vi "test_Delete FPGA Addon.vi"(8 "error in (no error)":errorcluster, 11 "TestCase in":refnum<class "FPGA Addon Scripting API Unit Tests.lvclass">) -> (0 "error out":errorcluster, 3 "TestCase out":refnum<class "FPGA Addon Scripting API Unit Tests.lvclass">)   [LabVIEW 2021, in "FPGA Addon Scripting API Unit Tests.lvclass"]
uses:
  FPGA Addon Scripting API Unit Tests.lvclass
  <vilib>/addons/_JKI Toolkits/VI Tester/TestCase.llb/TestCase.lvclass
  FPGA Addon Test Class/FPGA Addon Test Class.lvclass
  <vilib>/NI VeriStand/Custom Device Tools/Custom Device Utility Library/Custom Device Utility Library.lvlib
  APIs/Scripting API/Scripting API.lvlib
  C:/Program Files/National Instruments/LabVIEW 2021/vi.lib/addons/_JKI Toolkits/VI Tester/TestCase.llb/TestCase.lvclass
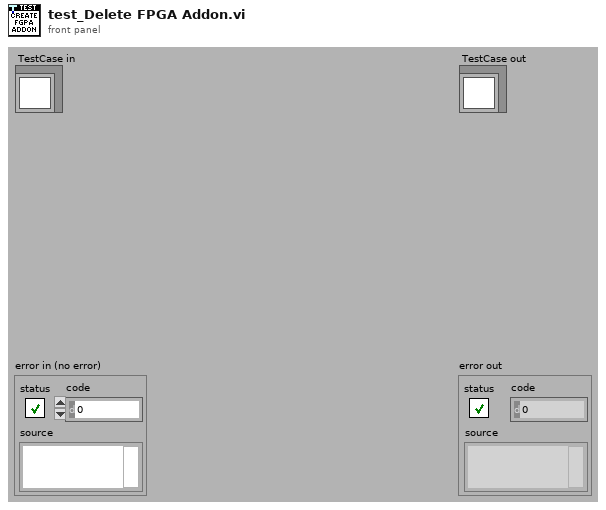
[diagram p1: front panel]
types:
  T1 = typedef "Custom Device API.lvlib/Custom Device Item Ref.ctl" = u64
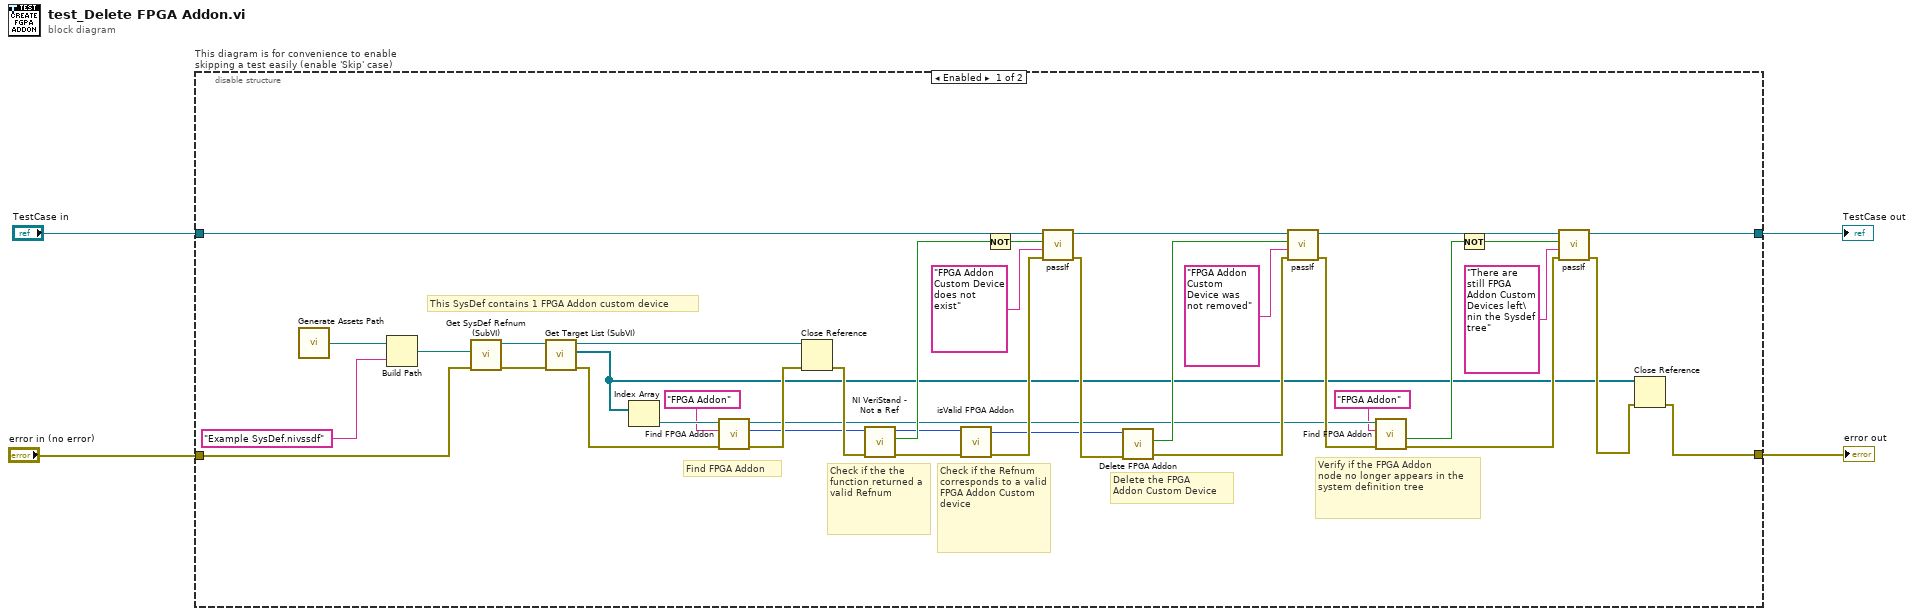
[diagram p0: block diagram]
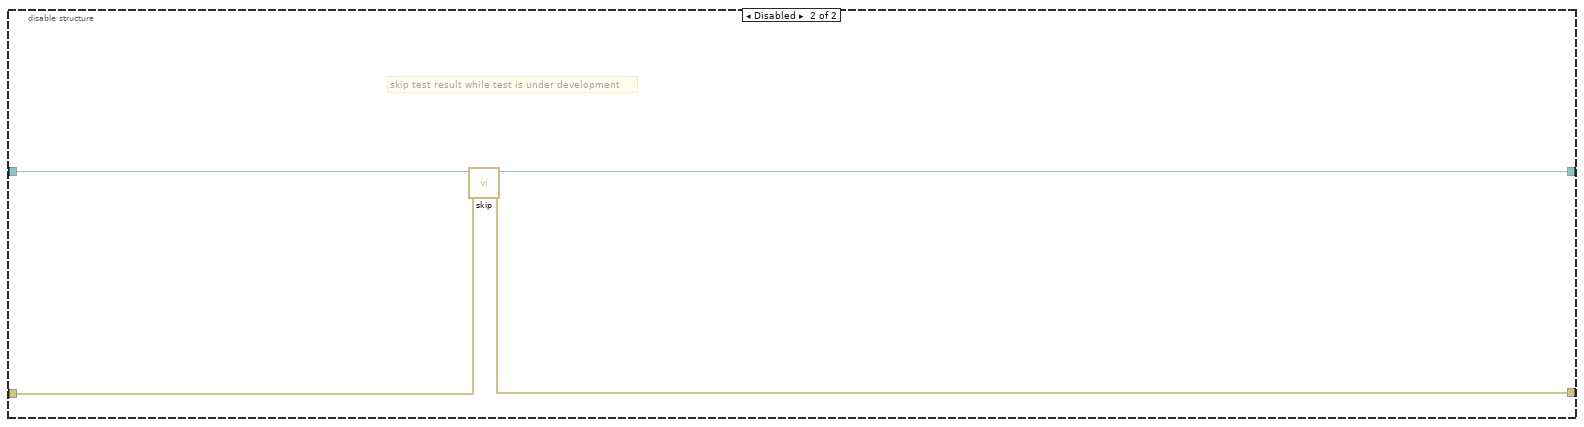
[diagram p2: hidden frame]
diagram:
  n1 = disable-structure "This diagram is for convenience to enable skipping a test easily (enable 'Skip' case)" shown="Enabled" {
    disable-tunnel: "TestCase in" -> [w36 w46]
    disable-tunnel: [w14 w44] -> w1
    disable-tunnel: [w6 w45] -> w3
    disable-tunnel: "error in (no error)" -> [w38 w43]
    frame Enabled {
      # "Verify if the FPGA Addon\nnode no longer appears in the \nsystem definition tree"
      # "Delete the FPGA \nAddon Custom Device"
      # "Check if the Refnum corresponds to a valid FPGA Addon Custom device"
      # "Check if the the function returned a valid Refnum"
      # "This SysDef contains 1 FPGA Addon custom device"
      # "Find FPGA Addon"
      n2 = call "Generate Assets Path.vi"() -> ("Assets path"=w42:path)
      n3 = Build Path(base path=w42, name or relative path="Example SysDef.nivssdf") -> (appended path=w40:path)
      n4 = call "Get SysDef Refnum (SubVI).vi"("error in (no error)"=w38, "System Definition path"=w40) -> ("error out"=w37:errorcluster, "SysDef Refnum out"=w39:refnum<k24>)  [unwired: 8 in]
      n5 = call "Get Target List (SubVI).vi"("error in (no error)"=w37, "SysDef Refnum in"=w39) -> ("error out"=w27:errorcluster, "Target List Refnums"=w7:refnum<k24>[], "SysDef Refnum out"=w32:refnum<k24>)  [unwired: 7 in]
      n6 = Index Array(array=w7) -> (element=w25:refnum<k24>)  [unwired: 1 in]
      n7 = call "Find FPGA Addon.vi"("error in"=w27, "FPGA addon name"="FPGA Addon", "target in"=w25) -> ("error out"=w26:errorcluster, "FPGA addon refnum out"=w23:T1, "target out"=w10:refnum<k24>)  [unwired: 5 in, 1 out]
      n8 = Close Reference(reference=w32, error in (no error)=w26) -> (error out=w31:errorcluster)
      n9 = call <vilib>:"NI VeriStand - Not a Ref.vi"("error in (no error)"=w31, "Item Ref"=w23) -> ("error out"=w30:errorcluster, "Not a Ref"=w35:bool, "Item Ref out"=w29:T1)  [unwired: 7 in]
      n10 = call "isValid FPGA Addon.vi"("error in"=w30, "FPGA Addon refnum in"=w29) -> ("error out"=w28:errorcluster, "FPGA Addon refnum out"=w20:T1)  [unwired: 8 in]
      n11 = Not(x=w35) -> (.not. x?=w34:bool)
      n12 = call-dynamic "passIf.vi"("error in (no error)"=w28, "message (\"\")"="FPGA Addon Custom Device does not exist" ("message (\"\")"), "pass"=w34, "TestCase in"=w36) -> ("error out"=w21:errorcluster, "TestCase out"=w22:refnum<class "FPGA Addon Scripting API Unit Tests.lvclass">)  [unwired: 6 in]
      n13 = call "Delete FPGA Addon.vi"("error in"=w21, "FPGA addon refnum"=w20) -> ("error out"=w18:errorcluster, "Deleted?"=w19:bool)  [unwired: 8 in]
      n14 = call-dynamic "passIf.vi"("error in (no error)"=w18, "message (\"\")"="FPGA Addon Custom Device was not removed" ("message (\"\")"), "pass"=w19, "TestCase in"=w22) -> ("error out"=w13:errorcluster, "TestCase out"=w16:refnum<class "FPGA Addon Scripting API Unit Tests.lvclass">)  [unwired: 6 in]
      n15 = call "Find FPGA Addon.vi"("error in"=w13, "FPGA addon name"="FPGA Addon", "target in"=w10) -> ("error out"=w12:errorcluster, "found ?"=w11:bool)  [unwired: 5 in, 2 out]
      n16 = Not(x=w11) -> (.not. x?=w5:bool)
      n17 = call-dynamic "passIf.vi"("error in (no error)"=w12, "message (\"\")"="There are still FPGA Addon Custom Devices left\nin the Sysdef tree" ("message (\"\")"), "pass"=w5, "TestCase in"=w16) -> ("error out"=w8:errorcluster, "TestCase out"=w14:refnum<class "FPGA Addon Scripting API Unit Tests.lvclass">)  [unwired: 6 in]
      n18 = Close Reference(reference=w7, error in (no error)=w8) -> (error out=w6:errorcluster)
    }
    frame Disabled {
      # "skip test result while test is under development"
      n19 = call <vilib>:"skip.vi"("error in (no error)"=w43, "TestCase in"=w46) -> ("error out"=w45:errorcluster, "TestCase out"=w44:refnum<class "FPGA Addon Scripting API Unit Tests.lvclass">)  [unwired: 8 in]
    }
  }
  "error out" <- w3
  "TestCase out" <- w1
